vi "Init.vi"(9 "Team ID":T1 format="%.0x", 10 "Index":i32, 11 "Team in":refnum<class "Team.lvclass">) -> (3 "Team out":refnum<class "Team.lvclass">)   [LabVIEW 2020, in "SquareBattle.lvlib" / "Team.lvclass"]
uses:
  Team.lvclass
  Team ID.ctl
  Team.lvclass/Team.ctl
  SquareBattle.lvlib
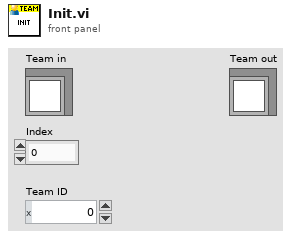
[diagram p1: front panel]
types:
  T1 = typedef "SquareBattle.lvlib/Team ID.ctl" = u32
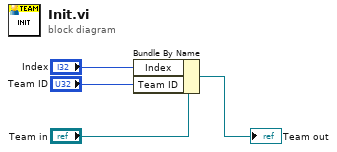
[diagram p0: block diagram]
diagram:
  n1 = Bundle By Name(cluster="Team in", "Index"="Index", "Team ID"="Team ID") -> (→"Team out":refnum<class "Team.lvclass">)
